vi "Wait - Copy-C.vi"(11 "Params":string[][](array[string])) -> ()   [LabVIEW 2017]
uses:
  RoutineData.vi
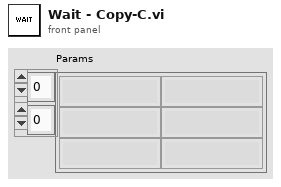
[diagram p1: front panel]
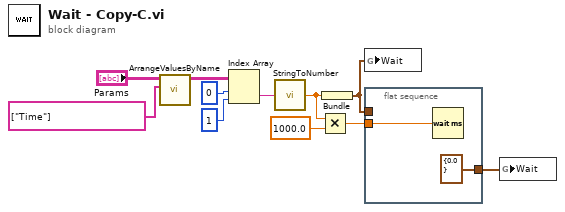
[diagram p0: block diagram]
diagram:
  n1 = call "ArrangeValuesByName.vi"("Names"=string[] ["Time"], "Names/Values in"="Params") -> ("Names/Values Out"=w4:string[][])  [unwired: 9 in]
  n2 = Index Array(array=w4, index (row)=0, index (col)=1) -> (element=w1:string)
  n3 = call "StringToNumber.vi"("String"=w1) -> ("Output"=w9:dbl)
  n4 = Multiply(x=w9, y=1000.0) -> (x*y=w7:dbl)
  n5 = Bundle("Output"=w9) -> (w11:cluster{"Output":dbl})  [unwired: 1 in]
  n6 = global write "RoutineData.vi" "Wait"(w11) -> ()
  n7 = flat-sequence {
    tunnel: w11 -> [_]
    tunnel: [cluster{"Distance":dbl} {"Distance"=0.0} ("output cluster")] -> w10
    tunnel: w7 -> [w12]
    frame #0 {
      n8 = Wait (ms)(milliseconds to wait=w12) -> ()  [unwired: 1 out]
    }
  }
  n9 = global write "RoutineData.vi" "Wait"(w10) -> ()
